vi "ConfigInstr.vi"(6 "InstrumentName":string, 7 "VisaRessIn":refnum<visa-resource-name>, 8 "error in (no error)":errorcluster caption="entrée d'erreur (pas d'erreur)", 9 "FirstClassInst":bool, 10 "Function":string, 11 "GenData In":refnum<class "SR830.lvclass"> caption="DNL_LabVIEW Object in") -> (0 "error out":errorcluster caption="sortie d'erreur", 3 "GenData Out":refnum<class "SR830.lvclass"> caption="DNL_LabVIEW Object out")   [LabVIEW 2019, in "SR830.lvclass"]
uses:
  SR830.lvclass
  C:/Programmes Labview/LabScanV1A/DevicesClass/BaseDevice/BaseDevice.lvclass
  SR830_Func.ctl
  SR830.lvclass/SR830.ctl
  BaseDevice/BaseDevice.lvclass/BaseDevice.ctl
  BaseDevice/Accessor/SetShowInstrNm.vi
panel:
  in  "Class_Func":T1
  out "VisaRessOut":refnum<visa-resource-name>
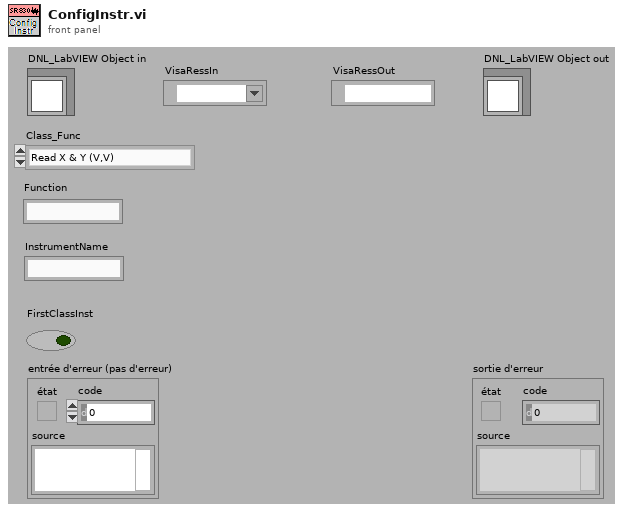
[diagram p1: front panel]
types:
  T1 = typedef "SR830.lvclass/SR830_Func.ctl" = enum16{"Read X & Y (V,V)", "Read Mag & Phase (V,°)", "Read X,Y,Mag & Phase (V,V,V,°)", "Read THz Pump Off/On (V,V,V,°,V,V,V,°,V)"}
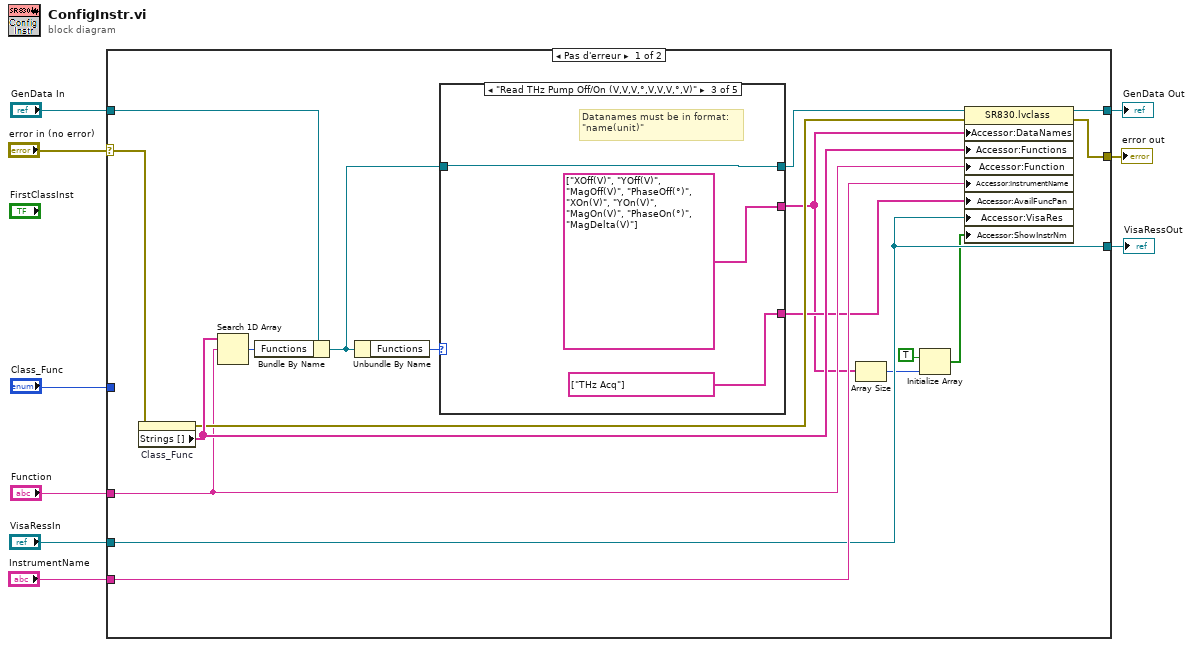
[diagram p0: block diagram]
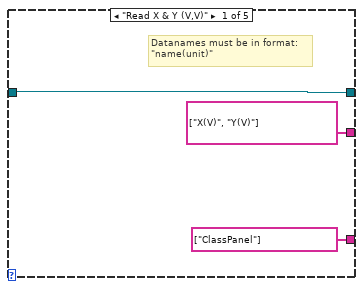
[diagram p2: hidden frame]
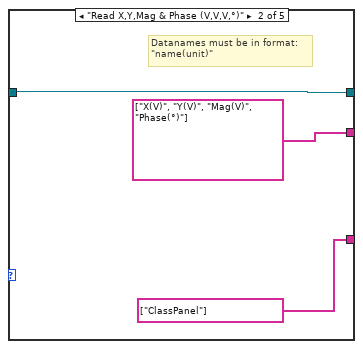
[diagram p3: hidden frame]
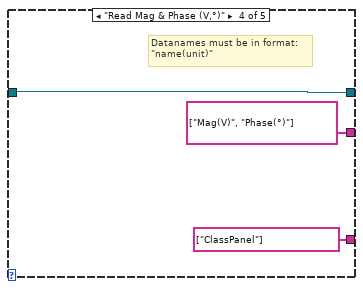
[diagram p4: hidden frame]
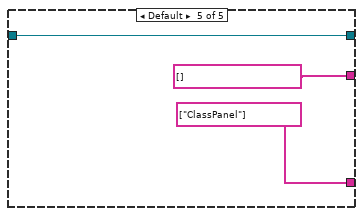
[diagram p5: hidden frame]
diagram:
  n1 = case shown="Pas d'erreur" "error in (no error)" {
    selector: "error in (no error)" -> [w21 w44]
    tunnel: [w27 w44] -> w8
    tunnel: "GenData In" -> [w22 w43]
    tunnel: [w26 w43] -> w6
    tunnel: "Class_Func" -> [_ _]
    tunnel: "Function" -> [w17 _]
    tunnel: "InstrumentName" -> [w16 _]
    tunnel: "VisaRessIn" -> [w14 _]
    tunnel: [w14 _] -> w1
    frame No Error {
      n2 = property on="Class_Func" class="Énum (strict)"(error in=w21) -> (error out=w20:errorcluster, "Strings []"=w24:string[])  [unwired: 1 in, 1 out]
      n3 = Search 1D Array(1D array=w24, element=w17) -> (index of element=w23:i32)  [unwired: 1 in]
      n4 = Bundle By Name(cluster=w22, "Functions"=w23) -> (w19:refnum<class "SR830.lvclass">)
      n5 = Unbundle By Name(w19) -> ("Functions"=w25:T1)
      n6 = case shown="\"Read THz Pump Off/On (V,V,V,°,V,V,V,°,V)\"" w25 {
        tunnel: [string[] ["X(V)", "Y(V)"] string[] ["X(V)", "Y(V)", "Mag(V)", "Phase(°)"] string[] ["XOff(V)", "YOff(V)", "MagOff(V)", "PhaseOff(°)", "XOn(V)", "YOn(V)", "MagOn(V)", "PhaseOn(°)", "MagDelta(V)"] string[] ["Mag(V)", "Phase(°)"] string[] []] -> w13
        tunnel: w19 -> [w30 w33 w36 w39 w41]
        tunnel: [w30 w33 w36 w39 w41] -> w18
        tunnel: [string[] ["ClassPanel"] string[] ["ClassPanel"] string[] ["THz Acq"] string[] ["ClassPanel"] string[] ["ClassPanel"]] -> w15
        frame "Read X & Y (V,V)" {
          # "Datanames must be in format:\n\"name(unit)\""
        }
        frame "Read X,Y,Mag & Phase (V,V,V,°)" {
          # "Datanames must be in format:\n\"name(unit)\""
        }
        frame "Read THz Pump Off/On (V,V,V,°,V,V,V,°,V)" {
          # "Datanames must be in format:\n\"name(unit)\""
        }
        frame "Read Mag & Phase (V,°)" {
          # "Datanames must be in format:\n\"name(unit)\""
        }
        frame Default {
        }
      }
      n7 = Array Size(array=w13) -> (size(s)=w12:i32)
      n8 = Initialize Array(TRUE, w12) -> (w10:bool[])
      n9 = property class="SR830.lvclass"(reference=w18, error in=w20, "Accessor:DataNames"=w13, "Accessor:Functions"=w24, "Accessor:Function"=w17, "Accessor:InstrumentName"=w16, "Accessor:AvailFuncPan"=w15, "Accessor:VisaRes"=w14, "Accessor:ShowInstrNm"=w10) -> (reference out=w26:refnum<class "SR830.lvclass">, error out=w27:errorcluster)
    }
    frame Error {
    }
  }
  "error out" <- w8
  "GenData Out" <- w6
  "VisaRessOut" <- w1
